vi "Joystick mapper.vi"(11 "Input":i32) -> (3 "Output":dbl)   [LabVIEW 2015, in "RDS Libraries.lvlib"]
uses:
  Geo/RDS Libraries.lvlib
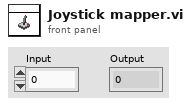
[diagram p1: front panel]
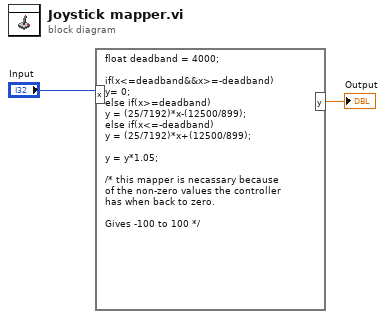
[diagram p0: block diagram]
diagram:
  n1 = formula code="float deadband = 4000;\n\nif(x<=deadband&&x>=-deadband)\ny= 0;\nelse if(x>=deadband)\ny = (25/7192)*x-(12500/899);\nelse if(x<=-deadband)\ny = (25/7192)*x+(12500/899);\n\ny = y*1.05;\n\n/* this mapper is necassary because\nof the non-zero values the controller\nhas when back to zero.\n\nGives -100 to 100 */"("x"="Input") -> ("y"=→"Output":dbl)
